vi "FTW-Socket-Destroy.vi"(0 "FTW Socket":refnum<class "FTW-Socket.lvclass">, 11 "error in":errorcluster) -> (15 "error out":errorcluster)   [LabVIEW 2013, in "FTW-Socket.lvclass"]
uses:
  FTW-Socket.lvclass
  FTW-Socket.lvclass/FTW-Socket.ctl
panel:
  # "Inputs"
  # "Outputs"
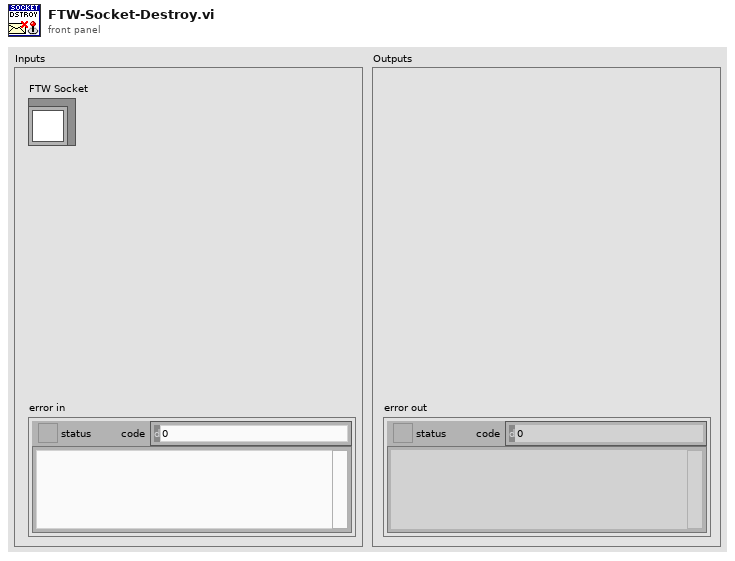
[diagram p1: front panel]
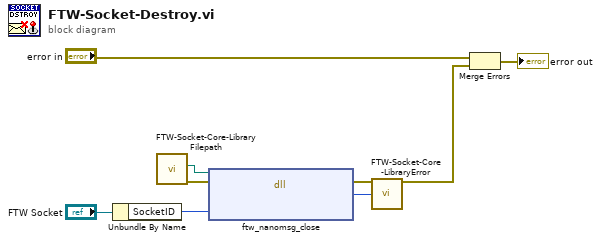
[diagram p0: block diagram]
diagram:
  n1 = Unbundle By Name("FTW Socket") -> ("SocketID"=w2:i64)
  n2 = call "FTW-Socket-Core-LibraryFilepath.vi"() -> ("error out"=w1:errorcluster, "Library Filepath"=w3:path)  [unwired: 9 in, 1 out]
  n3 = dll-call lib="?" fn="ftw_nanomsg_close"(path in=w3, error in=w1, "SocketID"=w2) -> (error out=w5:errorcluster, "Return Value"=w6:i64)  [unwired: 2 in, 1 out]
  n4 = call "FTW-Socket-Core-LibraryError.vi"("error in"=w5, "Return Value"=w6) -> ("error out"=w4:errorcluster)  [unwired: 13 in]
  n5 = Merge Errors("error in", w4) -> (→"error out":errorcluster)
